vi "Wojtyna_Target_C_2.vi"   [LabVIEW 2020]
uses:
  <vilib>/Platform/TimedLoop/XDataNode/timing_clust.ctl
  <vilib>/Platform/TimedLoop/XDataNode/nitl_modes.ctl
  <vilib>/Platform/TimedLoop/XDataNode/wakeup.ctl
  <vilib>/platform/TimedLoop/XDataNode/XDataNode.xnode
  <vilib>/Platform/TimedLoop/XDataNode/XDNodeRunTimeDep.lvlib
types:
  T1 = typedef "XDNodeRunTimeDep.lvlib/timing_clust.ctl" = cluster{"Expected End [f-1]":u64, "Actual End [f-1]":u64, "Finished Late? [f-1]":bool, "Expected End [i-1]":u64, "Actual End [i-1]":u64, "Finished Late? [i-1]":bool, "Expected Start [i]":u64, "Actual Start [i]":u64, "Expected Start [f]":u64, "Actual Start [f]":u64, "Source Name":string, "Structure Name":string, "Period":i64, "Deadline":i64, "Offset":i64, "Start":i64, "Priority":i32, "Timeout":i32, "Mode":T2, "Wakeup Reason":T3, "Error":errorcluster, "Source Type":string, "Secondary Source Type":string, "Global End Time":u64, "Global Start Time":u64, "Frame Duration":u64, "Iteration Duration":u64, "Assigned CPU":i32, "I/O Scan Engine Mode":u32}
  T2 = typedef "XDNodeRunTimeDep.lvlib/nitl_modes.ctl" = enum32{"No Change", "Process missed periods, maintain original phase", "Discard missed periods, maintain original phase", "Process missed periods, ignore original phase", "Discard missed periods, ignore original phase"}
  T3 = typedef "XDNodeRunTimeDep.lvlib/wakeup.ctl" = enum32{"Normal", "Aborted", "Asynchronous wakeup", "Timing source error", "Timed loop error", "Timeout"}
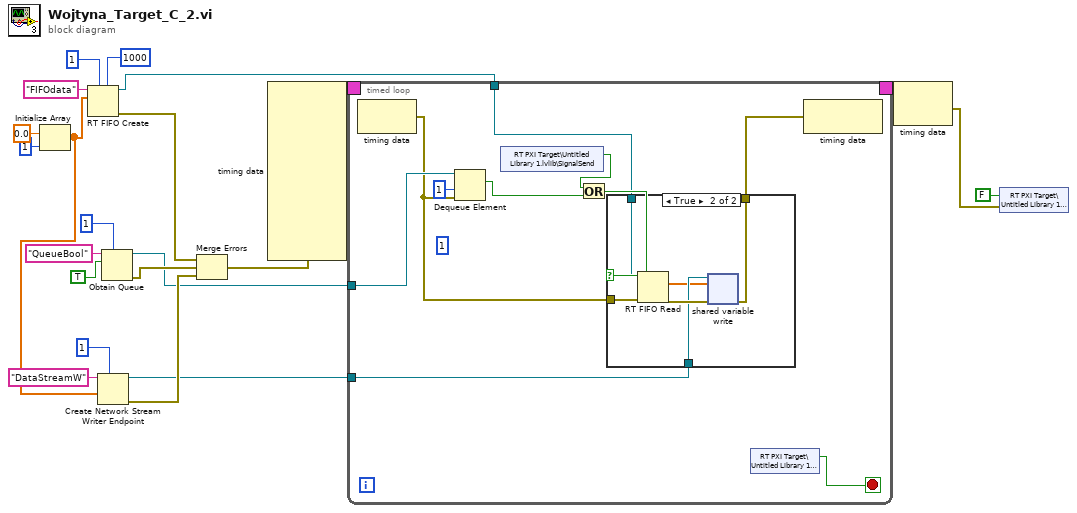
[diagram p0: block diagram]
diagram:
  n1 = Initialize Array(0.0 ("element"), 1 ("dimension size")) -> (w11:dbl[])
  n2 = RT FIFO Create(0:"FIFOdata" ("name (unnamed)"), 1:w11, 4:u32 1 ("size (10)"), 6:u32 1000 ("elements in array (1)")) -> (8:w4:refnum<k33>, 11:w9:errorcluster)  [unwired: 4 in, 1 out]
  n3 = Create Network Stream Writer Endpoint(7:1 ("writer buffer size"), 9:w11, 11:"DataStreamW" ("writer name")) -> (0:w7:errorcluster, 3:w3:refnum<k21>)  [unwired: 4 in]
  n4 = Obtain Queue(max queue size (-1, unlimited)=1, name (unnamed)="QueueBool", element data type=TRUE) -> (queue out=w5:refnum<queue>, error out=w8:errorcluster)  [unwired: 2 in, 1 out]
  n5 = Merge Errors(w9, w8, w7) -> (w6:errorcluster)
  n6 = node-c288(w6) -> (w22:T1)  [unwired: 9 in]
  n7 = timed-loop {
    timing: w22 -> [_]
    timing-out: [_] -> w21
    tunnel: w5 -> [w31]
    tunnel: w4 -> [w28]
    tunnel: w3 -> [w26]
    stop <- w25 stop-if-true
    (unwired) 1 ("timeout in ms (0)")
    n8 = node-c288() -> (w27:errorcluster)  [unwired: 1 in]
    n9 = Dequeue Element(queue=w31, timeout in ms (-1)=1, error in (no error)=w27) -> (element=w30:bool)  [unwired: 3 out]
    n10 = shared-variable "RT PXI Target\\Untitled Library 1.lvlib\\SignalSend"() -> (w23:bool)  [unwired: 1 in, 1 out]
    n11 = Or(x=w23, y=w30) -> (x .or. y?=w29:bool)
    n12 = case shown="True" w29 {
      tunnel: w28 -> [_ w39]
      tunnel: w27 -> [w33 w38]
      tunnel: w26 -> [_ w36]
      tunnel: [w33 w34] -> w24
      frame False {
      }
      frame True {
        n13 = RT FIFO Read(0:w39, 3:w38) -> (9:w35:dbl[], 11:w37:errorcluster)  [unwired: 2 in, 3 out]
        n14 = shared-variable-write(w36, w37, w35) -> (w34:errorcluster)  [unwired: 1 in, 2 out]
      }
    }
    n15 = shared-variable "RT PXI Target\\Untitled Library 1.lvlib\\Stop"() -> (w25:bool)  [unwired: 1 in, 1 out]
    n16 = node-c288(w24) -> ()  [unwired: 1 out]
  }
  n17 = node-c288(w21) -> (w2:errorcluster)
  n18 = shared-variable "RT PXI Target\\Untitled Library 1.lvlib\\Stop"(FALSE ("Stop"), error in=w2) -> ()  [unwired: 1 out]
